vi "Read Rolebook.vi"(8 "error in (no error)":errorcluster, 11 "Play in":refnum<class "Play.lvclass">) -> (0 "error out":errorcluster, 2 "Rolebook":refnum<class "Rolebook.lvclass">, 3 "Play out":refnum<class "Play.lvclass">)   [LabVIEW 2023, in "Play.lvclass"]
uses:
  Play.lvclass
  Rolebook_class/Rolebook.lvclass
  Play.lvclass/Play.ctl
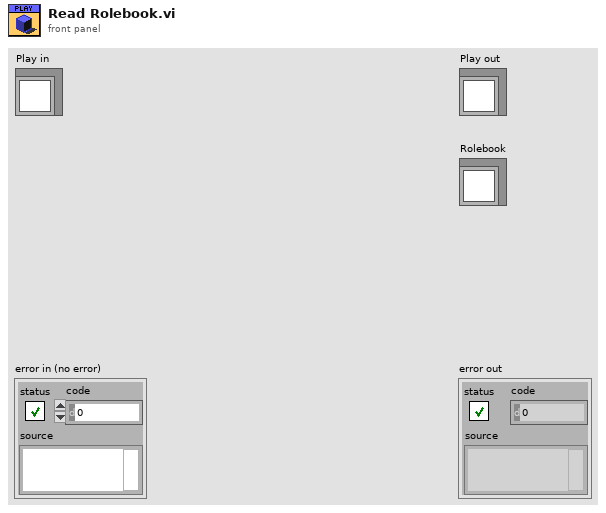
[diagram p1: front panel]
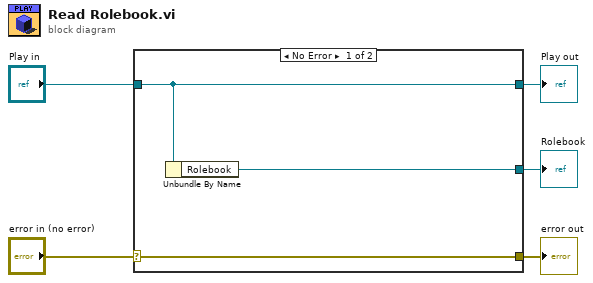
[diagram p0: block diagram]
diagram:
  n1 = case shown="No Error" "error in (no error)" {
    selector: "error in (no error)" -> [w8 w9]
    tunnel: [w8 w9] -> w4
    tunnel: [w7 w10] -> w2
    tunnel: "Play in" -> [w7 w10]
    tunnel: [w6 _] -> w1
    frame No Error {
      n2 = Unbundle By Name(w7) -> ("Rolebook"=w6:refnum<class "Rolebook.lvclass">)
    }
    frame Error {
    }
  }
  "error out" <- w4
  "Play out" <- w2
  "Rolebook" <- w1
